vi "create_class_items.vi"(8 "error in":errorcluster, 10 "item creation flags":T1, 11 "new class reference in":refnum<vi>) -> (0 "error out":errorcluster, 3 "new class reference out":refnum<vi>)   [LabVIEW 2010]
uses:
  item_creation_flags_cluster.ctl
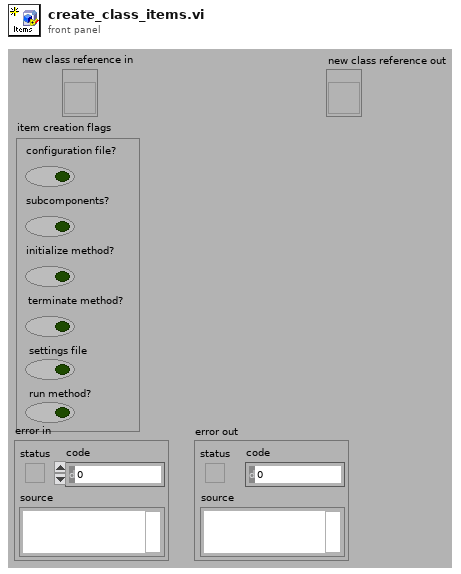
[diagram p1: front panel]
types:
  T1 = typedef "item_creation_flags_cluster.ctl" = cluster{"configuration file?":bool, "subcomponents?":bool, "initialize method?":bool, "terminate method?":bool, "settings file":bool, "run method?":bool}
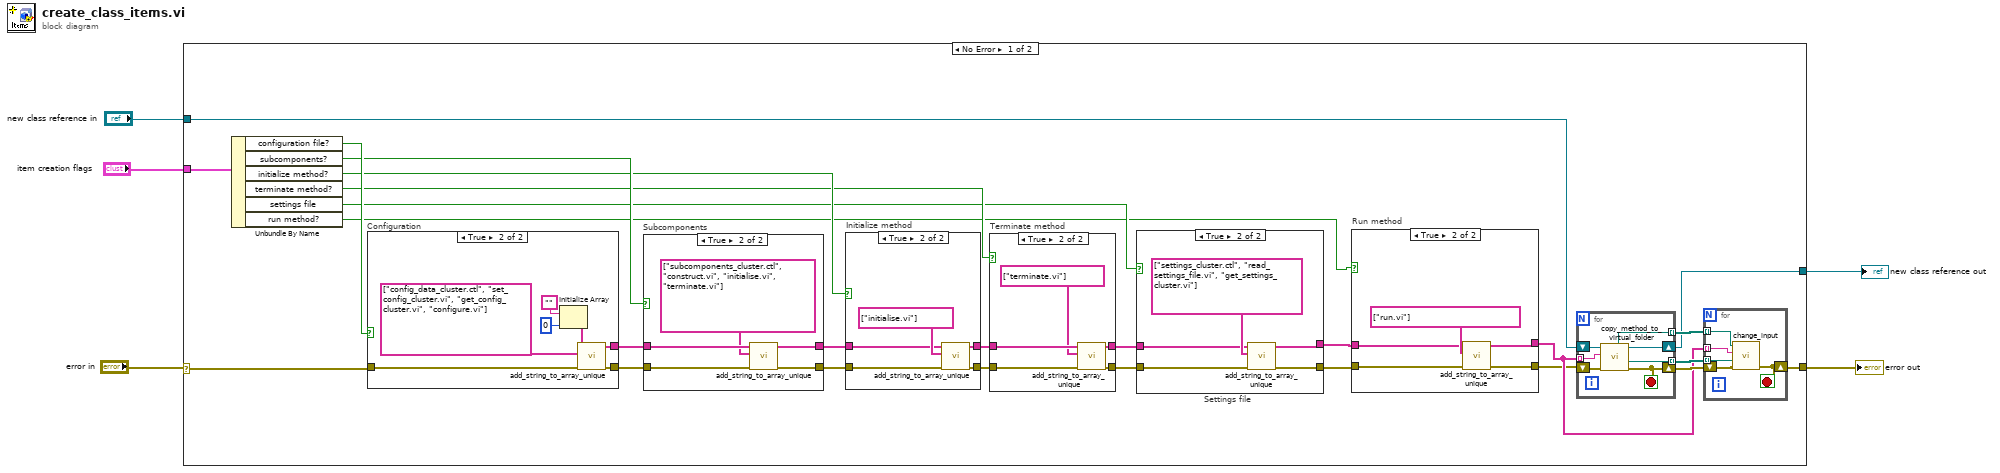
[diagram p0: block diagram]
diagram:
  n1 = case shown="No Error" "error in" {
    selector: "error in" -> [w13 w88]
    tunnel: "item creation flags" -> [w31 _]
    tunnel: [w14 w88] -> w4
    tunnel: [w12 w87] -> w2
    tunnel: "new class reference in" -> [w11 w87]
    frame No Error {
      n2 = Unbundle By Name(w31) -> ("configuration file?"=w30:bool, "subcomponents?"=w29:bool, "initialize method?"=w28:bool, "terminate method?"=w27:bool, "settings file"=w26:bool, "run method?"=w10:bool)
      n3 = case "Configuration" shown="True" w30 {
        tunnel: [_ w82] -> w24
        tunnel: [w79 w81] -> w25
        tunnel: w13 -> [w79 w80]
        frame False {
        }
        frame True {
          n4 = Initialize Array("", 0 ("dimension size")) -> (w83:string[])
          n5 = call "add_string_to_array_unique.vi"("error in (no error)"=w80, "strings to add"=string[] ["config_data_cluster.ctl", "set_config_cluster.vi", "get_config_cluster.vi", "configure.vi"], "array in"=w83) -> ("error out"=w81:errorcluster, "array out"=w82:string[])  [unwired: 7 in]
        }
      }
      n6 = case "Subcomponents" shown="True" w29 {
        tunnel: w25 -> [w66 w71]
        tunnel: [w66 w67] -> w23
        tunnel: w24 -> [w65 w70]
        tunnel: [w65 w68] -> w22
        frame False {
        }
        frame True {
          n7 = call "add_string_to_array_unique.vi"("error in (no error)"=w71, "strings to add"=string[] ["subcomponents_cluster.ctl", "construct.vi", "initialise.vi", "terminate.vi"], "array in"=w70) -> ("error out"=w67:errorcluster, "array out"=w68:string[])  [unwired: 7 in]
        }
      }
      n8 = case "Initialize method" shown="True" w28 {
        tunnel: w23 -> [w58 w64]
        tunnel: [w58 w63] -> w20
        tunnel: [w59 w62] -> w21
        tunnel: w22 -> [w59 w60]
        frame False {
        }
        frame True {
          n9 = call "add_string_to_array_unique.vi"("error in (no error)"=w64, "strings to add"=string[] ["initialise.vi"], "array in"=w60) -> ("error out"=w63:errorcluster, "array out"=w62:string[])  [unwired: 7 in]
        }
      }
      n10 = case "Terminate method" shown="True" w27 {
        tunnel: w21 -> [w52 w57]
        tunnel: w20 -> [w51 w56]
        tunnel: [w52 w53] -> w19
        tunnel: [w51 w54] -> w18
        frame False {
        }
        frame True {
          n11 = call "add_string_to_array_unique.vi"("error in (no error)"=w56, "strings to add"=string[] ["terminate.vi"], "array in"=w57) -> ("error out"=w54:errorcluster, "array out"=w53:string[])  [unwired: 7 in]
        }
      }
      n12 = case "Settings file" shown="True" w26 {
        tunnel: w19 -> [w44 w49]
        tunnel: w18 -> [w45 w48]
        tunnel: [w44 w47] -> w8
        tunnel: [w45 w46] -> w7
        frame False {
        }
        frame True {
          n13 = call "add_string_to_array_unique.vi"("error in (no error)"=w48, "strings to add"=string[] ["settings_cluster.ctl", "read_settings_file.vi", "get_settings_cluster.vi"], "array in"=w49) -> ("error out"=w46:errorcluster, "array out"=w47:string[])  [unwired: 7 in]
        }
      }
      n14 = case "Run method" shown="True" w10 {
        tunnel: w8 -> [w33 w37]
        tunnel: w7 -> [w32 w36]
        tunnel: [w33 w35] -> w9
        tunnel: [w32 w34] -> w6
        frame False {
        }
        frame True {
          n15 = call "add_string_to_array_unique.vi"("error in (no error)"=w36, "strings to add"=string[] ["run.vi"], "array in"=w37) -> ("error out"=w34:errorcluster, "array out"=w35:string[])  [unwired: 7 in]
        }
      }
      n16 = for {
        shift-right: [w72] -> w15
        shift-left: w6 -> [w78]
        shift-right: [w77] -> w12
        shift-left: w11 -> [w76]
        tunnel: w9 -> [w75] mode=indexing
        tunnel: [w74] -> w17 mode=indexing
        tunnel: [w73] -> w16 mode=indexing
        stop <- w72 stop-if-true
        n17 = call "copy_method_to_virtual_folder.vi"("error in"=w78, "name or relative path"=w75, "new class reference in"=w76) -> ("error out"=w72:errorcluster, "new vi path out"=w73:path, "new class reference out"=w77:refnum<vi>, "new class path out"=w74:path)  [unwired: 5 in]
      }
      n18 = for {
        tunnel: w17 -> [w43] mode=indexing
        tunnel: w16 -> [w42] mode=indexing
        shift-right: [w39] -> w14
        shift-left: w15 -> [w41]
        tunnel: w9 -> [w40] mode=indexing
        stop <- w39 stop-if-true
        n19 = call "change_input.vi"("error in"=w41, "new vi path in"=w42, "name or relative path in"=w40, "new class path in"=w43) -> ("error out"=w39:errorcluster)  [unwired: 7 in]
      }
    }
    frame Error {
    }
  }
  "error out" <- w4
  "new class reference out" <- w2
